vi "ConfigureRF.vi"(8 "error in (no error)":errorcluster, 11 "reference in":refnum<class "sim_MmW.lvclass">) -> (0 "error out":errorcluster, 3 "reference out":refnum<class "sim_MmW.lvclass">)   [LabVIEW 2019, in "sim_MmW.lvclass"]
doc: "Configures RF setting at specified port:\n<b>Frequency</b> - operating frequency (RF/IF)\n<b>Gain</b> - Signal gain"
uses:
  sim_MmW.lvclass
  C:/Barkhausen mmWave radar/Development/modules/mmw_instrument/src_LabVIEW/Host/SubVIs/mmWave instrument_class/mmWave instrument.lvclass
  Low-level/TypeDefs/Front End Configuration.ctl
  Low-level/TypeDefs/Channel Configuration.ctl
  <instrlib>/niMmWave/ni3620/Config/v1/Host/Public/Typedefs/mmWave Port.ctl
  mmWave instrument_class/mmWave instrument.lvclass
  <instrlib>/niMmWave/ni3620/Config/v1/Host/niMmWave Config v1 Host.lvlib
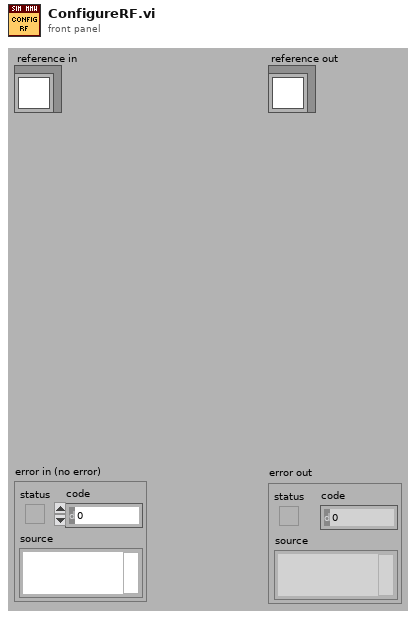
[diagram p1: front panel]
types:
  T1 = typedef "niMmWave Config v1 Host.lvlib/mmWave Port.ctl" = string
  T2 = typedef "Front End Configuration.ctl" = cluster{"port select":enum16{"IF Port", "Loopback", "Sync Port"}, "Rx hardware configuration":T3, "Tx hardware configuration":T3}
  T3 = typedef "Channel Configuration.ctl" = cluster{"gain (dB)":dbl, "frequency (Hz)":dbl, "mmWave adapter":string, "adapter active port":T1}
  T4 = typedef "sim_MmW.lvclass/ObjectAttributesRef.ctl" = refnum<data-value>
  T5 = typedef "mmWave instrument.lvclass/ObjectAttributes.ctl" = cluster{"mode":T6, "instr state":T7, "Max Fs":dbl, "Equalization coeff":cdb[], "LO sync en":bool, "Trig sync en":bool, "LO sources":T8, "LO Export":T9, "Fc.range":cluster{"min":dbl, "max":dbl}, "Sync mode":T10, "equalization en":bool, "sequence":string[]}
  T6 = typedef "mmWave instrument.lvclass/Instrument mode.ctl" = enum16{"RF", "IF", "BB"}
  T7 = typedef "mmWave instrument.lvclass/Instrument state.ctl" = enum16{"Off", "Initialization", "Configuration", "Running", "Calibration"}
  T8 = typedef "mmWave HW Control.lvlib/LO sources.ctl" = cluster{"RX/LO1 src":string, "TX/LO1 src":string, "LO2 src":string}
  T9 = typedef "mmWave HW Control.lvlib/LO export.ctl" = cluster{"TX LO1 export":bool, "TX LO1 export level":dbl, "RX LO1 export":bool, "RX LO1 export level":dbl, "LO2 export":bool, "LO2 export level":dbl}
  T10 = typedef "mmWave instrument.lvclass/Sync mode.ctl" = enum16{"Slave", "Master"}
  T11 = typedef "sim_MmW.lvclass/ObjectAttributes.ctl" = cluster{"RF config":T12, "RX samples":i32, "Downloaded Bursts":map{string, refnum<class "mmWave data.lvclass">}, "TX Fs":dbl, "RX Fs":dbl, "burst sequence":string[], "Burst mode":T13}
  T12 = typedef "mmWave HW Control.lvlib/HW TXRX RF config cluster.ctl" = cluster{"TX.Frequency":dbl, "TX.Gain":dbl, "TX.mmWave adapter":string, "RX.Frequency":dbl, "RX.Gain":dbl, "RX.mmWave adapter":string}
  T13 = typedef "mmWave instrument.lvclass/BurstMode.ctl" = enum16{"burst", "continuous"}
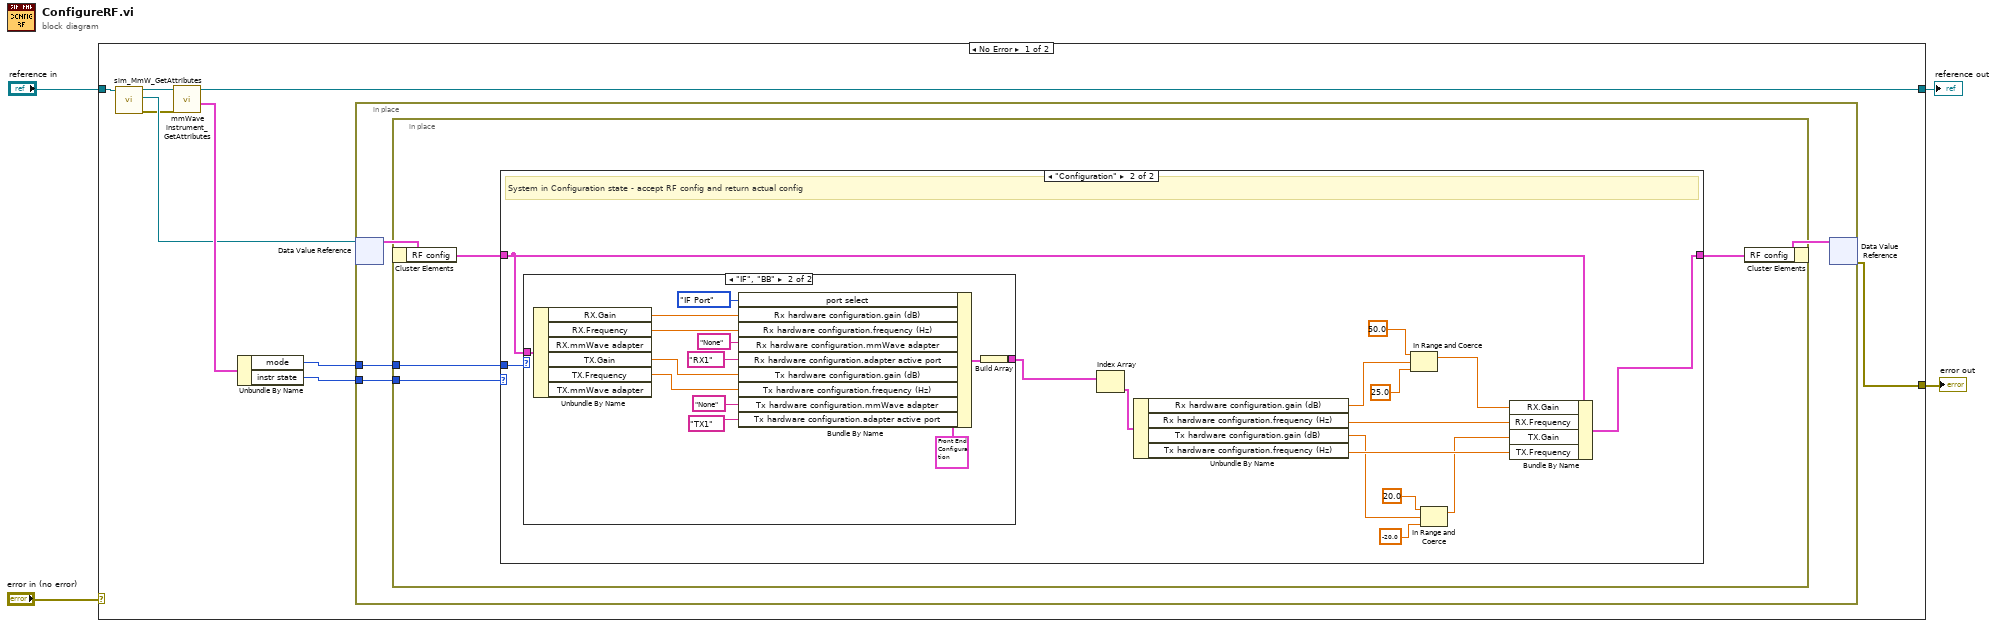
[diagram p0: block diagram]
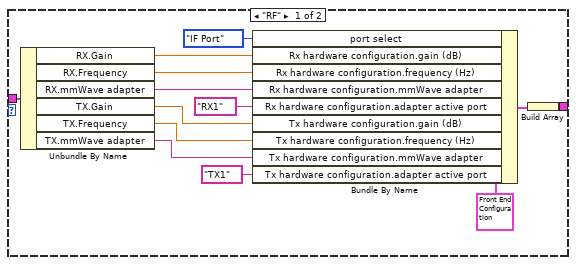
[diagram p3: hidden frame]
diagram:
  n1 = case shown="No Error" "error in (no error)" {
    selector: "error in (no error)" -> [_ w65]
    tunnel: [w5 w65] -> w3
    tunnel: [w11 w64] -> w1
    tunnel: "reference in" -> [w12 w64]
    frame No Error {
      n2 = call "sim_MmW_GetAttributes.vi"("reference in"=w12) -> ("error out"=w8:errorcluster, "attributes ref"=w9:T4, "reference out"=w13:refnum<class "sim_MmW.lvclass">)  [unwired: 7 in, 1 out]
      n3 = call "mmWave instrument_GetAttributes.vi"("error in (no error)"=w8, "reference in"=w13) -> ("attributes"=w10:T5, "reference out"=w11:refnum<class "sim_MmW.lvclass">)  [unwired: 6 in, 2 out]
      n4 = Unbundle By Name(w10) -> ("mode"=w7:T6, "instr state"=w6:T7)
      n5 = in-place {
        in-place-border: w7 -> [w15]
        in-place-border: w6 -> [w14]
        n6 = in-place-dvr #1(w9) -> (w17:T11)  [unwired: 1 out]
        n7 = in-place {
          in-place-border: w15 -> [w21]
          in-place-border: w14 -> [w19]
          n8 = in-place-cluster #2(w17) -> ("RF config"=w18:T12)
          n9 = case shown="\"Configuration\"" w19 {
            tunnel: w21 -> [_ w36]
            tunnel: [w22 w32] -> w20
            tunnel: w18 -> [w22 w31]
            frame "Off", Default {
            }
            frame "Configuration" {
              # "System in Configuration state - accept RF config and return actual config"
              n10 = case shown="\"IF\", \"BB\"" w36 {
                tunnel: [w50 w63] -> w37
                tunnel: w31 -> [w44 w58]
                frame "RF" {
                  n11 = Unbundle By Name(w44) -> ("RX.Gain"=w43:dbl, "RX.Frequency"=w42:dbl, "RX.mmWave adapter"=w41:string, "TX.Gain"=w40:dbl, "TX.Frequency"=w39:dbl, "TX.mmWave adapter"=w38:string)
                  n12 = Bundle By Name(cluster=T2 {"port select"=enum."Loopback", "Rx hardware configuration"={"gain (dB)"=15.0, "frequency (Hz)"=12000000000.0, "mmWave adapter"="None", "adapter active port"=""}, "Tx hardware configuration"={"gain (dB)"=-15.0, "frequency (Hz)"=12000000000.0, "mmWave adapter"="None", "adapter active port"=""}} ("device configuration [channel]"), "port select"=enum16{"IF Port", "Loopback", "Sync Port"}."IF Port", "Rx hardware configuration.gain (dB)"=w43, "Rx hardware configuration.frequency (Hz)"=w42, "Rx hardware configuration.mmWave adapter"=w41, "Rx hardware configuration.adapter active port"=T1 "RX1", "Tx hardware configuration.gain (dB)"=w40, "Tx hardware configuration.frequency (Hz)"=w39, "Tx hardware configuration.mmWave adapter"=w38, "Tx hardware configuration.adapter active port"=T1 "TX1") -> (w49:T2)
                  n13 = Build Array(w49) -> (w50:T2[])
                }
                frame "IF", "BB" {
                  n14 = Unbundle By Name(w58) -> ("RX.Gain"=w57:dbl, "RX.Frequency"=w56:dbl, "TX.Gain"=w55:dbl, "TX.Frequency"=w54:dbl)  [unwired: 2 out]
                  n15 = Bundle By Name(cluster=T2 {"port select"=enum."Loopback", "Rx hardware configuration"={"gain (dB)"=15.0, "frequency (Hz)"=12000000000.0, "mmWave adapter"="None", "adapter active port"=""}, "Tx hardware configuration"={"gain (dB)"=-15.0, "frequency (Hz)"=12000000000.0, "mmWave adapter"="None", "adapter active port"=""}} ("device configuration [channel]"), "port select"=enum16{"IF Port", "Loopback", "Sync Port"}."IF Port", "Rx hardware configuration.gain (dB)"=w57, "Rx hardware configuration.frequency (Hz)"=w56, "Rx hardware configuration.mmWave adapter"="None", "Rx hardware configuration.adapter active port"=T1 "RX1", "Tx hardware configuration.gain (dB)"=w55, "Tx hardware configuration.frequency (Hz)"=w54, "Tx hardware configuration.mmWave adapter"="None" ("Rx hardware configuration.mmWave adapter"), "Tx hardware configuration.adapter active port"=T1 "TX1") -> (w62:T2)
                  n16 = Build Array(w62) -> (w63:T2[])
                }
              }
              n17 = Index Array(array=w37) -> (element=w35:T2)  [unwired: 1 in]
              n18 = Unbundle By Name(w35) -> ("Rx hardware configuration.gain (dB)"=w30:dbl, "Rx hardware configuration.frequency (Hz)"=w34:dbl, "Tx hardware configuration.gain (dB)"=w26:dbl, "Tx hardware configuration.frequency (Hz)"=w33:dbl)
              n19 = In Range and Coerce(upper limit=50.0 ("lower limit"), x=w30, lower limit=25.0) -> (coerced(x)=w27:dbl)  [unwired: 1 out]
              n20 = In Range and Coerce(upper limit=20.0 ("x"), x=w26, lower limit=-20.0 ("x")) -> (coerced(x)=w23:dbl)  [unwired: 1 out]
              n21 = Bundle By Name(cluster=w31, "RX.Gain"=w27, "RX.Frequency"=w34, "TX.Gain"=w23, "TX.Frequency"=w33) -> (w32:T12)
            }
          }
          n22 = in-place-cluster #2("RF config"=w20) -> (w16:T11)
        }
        n23 = in-place-dvr #1(w16) -> (w5:errorcluster)  [unwired: 1 out]
      }
    }
    frame Error {
    }
  }
  "error out" <- w3
  "reference out" <- w1
